vi "Set_Parameter_Instrument (Json).vi"(8 "error in (no error)":errorcluster caption="entrée d'erreur (pas d'erreur)", 10 "Parameter (Json)":string, 11 "Enable_DIO en entrée":refnum<class "Enable_DIO.lvclass">) -> (0 "error out":errorcluster caption="sortie d'erreur", 3 "Enable_DIO en sortie":refnum<class "Enable_DIO.lvclass">)   [LabVIEW 2020, in "Library Test.lvlib" / "Enable_DIO.lvclass"]
uses:
  Enable_DIO.lvclass
  C:/Users/ngarcin/OneDrive - Altyor/Standard TB/Class/Test/Test (Default)/Test (Default).lvclass
  Commun VI/TypeDef/Commande DIO/Parameter DIO.ctl
  DIO/Class DIO (Default)/Class DIO (Default).lvclass
  JSON API/JSON Value/Set from JSON string.vi
  JSON API/Variant JSON/Variant to JSON.vi
  JSON API/JSON Value/Get Item by name array.vi
  Test_Wtih_Instr/Test_With_Inst.lvclass
  Instrument/Instrument (Default)/Class Instrument (Default).lvclass
  JSON API/JSON Value/JSON Value.lvclass
  Enable_DIO.lvclass/Enable_DIO.ctl
  JSON API/Variant JSON/Variant JSON.lvlib
  JSON API/Get Polymorphic/JSON GetSet.lvlib
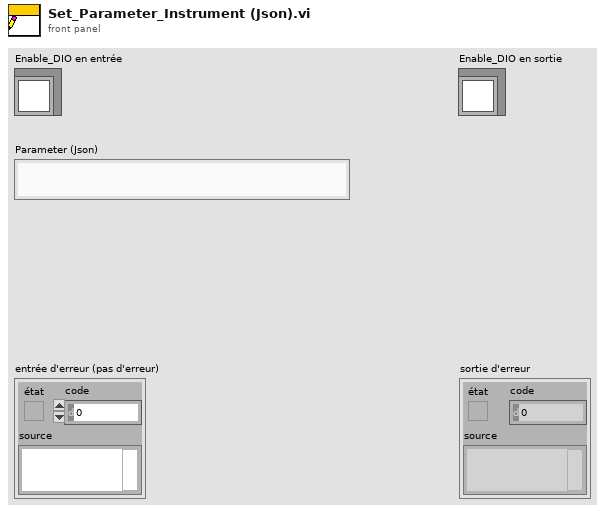
[diagram p1: front panel]
types:
  T1 = typedef "Parameter DIO.ctl" = cluster{"Device_Com_Port":string, "Port":u8, "Line":u8, "Function":enum16{"Write", "Read"}, "Class DIO":refnum<class "Class DIO (Default).lvclass">}
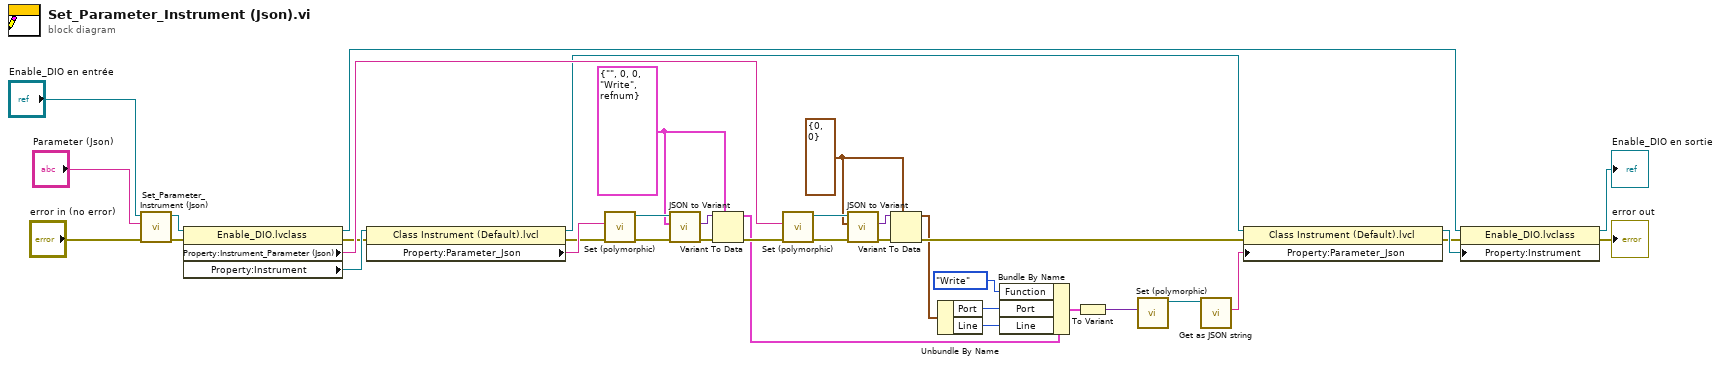
[diagram p0: block diagram]
diagram:
  w11 = T1 {"Device_Com_Port"="", "Port"=0, "Line"=0, "Function"=enum."Write", "Class DIO"=refnum} ("Parameter")
  w10 = cluster{"Line":u8, "Port":u8} {"Line"=0, "Port"=0} ("Cluster des données privées de classe")
  n1 = call-parent "Set_Parameter_Instrument (Json).vi"("error in (no error)"="error in (no error)", "Parameter (Json)"="Parameter (Json)", "Test (Default) en entrée"="Enable_DIO en entrée") -> ("error out"=w4:errorcluster, "Test (Default) en sortie"=w19:refnum<class "Enable_DIO.lvclass">)  [unwired: 7 in]
  n2 = property class="Enable_DIO.lvclass"(reference=w19, error in=w4) -> (reference out=w15:refnum<class "Enable_DIO.lvclass">, error out=w3:errorcluster, "Property:Instrument_Parameter (Json)"=w17:string, "Property:Instrument"=w18:refnum<class "Class Instrument (Default).lvclass">)
  n3 = property class="Class Instrument (Default).lvcl"(reference=w18, error in=w3) -> (reference out=w14:refnum<class "Class Instrument (Default).lvclass">, error out=w24:errorcluster, "Property:Parameter_Json"=w26:string)
  n4 = call-poly "Set (polymorphic).vi"("error in (no error)"=w24, "JSON stream"=w26) -> ("error out"=w28:errorcluster, "JSON Value out"=w30:refnum<class "JSON Value.lvclass">)  [unwired: 7 in, 1 out]
  n5 = call "JSON to Variant.vi"("error in (no error)"=w28, "Variant (Data Type)"=w11, "JSON Value"=w30) -> ("error out"=w29:errorcluster, "Variant out"=w27:variant)  [unwired: 7 in]
  n6 = Variant To Data(error in=w29, type=w11, Variant=w27) -> (data=w9:T1, error out=w25:errorcluster)
  n7 = call-poly "Set (polymorphic).vi"("error in (no error)"=w25, "JSON stream"=w17) -> ("error out"=w33:errorcluster, "JSON Value out"=w31:refnum<class "JSON Value.lvclass">)  [unwired: 7 in, 1 out]
  n8 = call "JSON to Variant.vi"("error in (no error)"=w33, "Variant (Data Type)"=w10, "JSON Value"=w31) -> ("error out"=w32:errorcluster, "Variant out"=w34:variant)  [unwired: 7 in]
  n9 = Variant To Data(error in=w32, type=w10, Variant=w34) -> (data=w7:cluster{"Line":u8, "Port":u8}, error out=w23:errorcluster)
  n10 = Unbundle By Name(w7) -> ("Port"=w6:u8, "Line"=w5:u8)
  n11 = Bundle By Name(cluster=w9, "Function"=enum16{"Write", "Read"}."Write", "Port"=w6, "Line"=w5) -> (w8:T1)
  n12 = To Variant(anything=w8) -> (Variant=w21:variant)
  n13 = call-poly "Set (polymorphic).vi"("Variant"=w21) -> ("JSON Value out"=w22:refnum<class "JSON Value.lvclass">)  [unwired: 9 in, 1 out]
  n14 = call "Get as JSON string.vi"("JSON Value in"=w22) -> ("<JSON>"=w20:string)  [unwired: 9 in, 1 out]
  n15 = property class="Class Instrument (Default).lvcl"(reference=w14, error in=w23, "Property:Parameter_Json"=w20) -> (reference out=w16:refnum<class "Class Instrument (Default).lvclass">, error out=w2:errorcluster)
  n16 = property class="Enable_DIO.lvclass"(reference=w15, error in=w2, "Property:Instrument"=w16) -> (reference out=→"Enable_DIO en sortie":refnum<class "Enable_DIO.lvclass">, error out=→"error out":errorcluster)
